vi "ECEF_2_LLA2(SubVI).vi"(11 "p_new":dbl[](array[numeric])) -> (1 "lon":dbl, 2 "latd":dbl, 3 "altd":dbl)   [LabVIEW 2017]
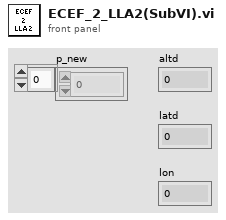
[diagram p1: front panel]
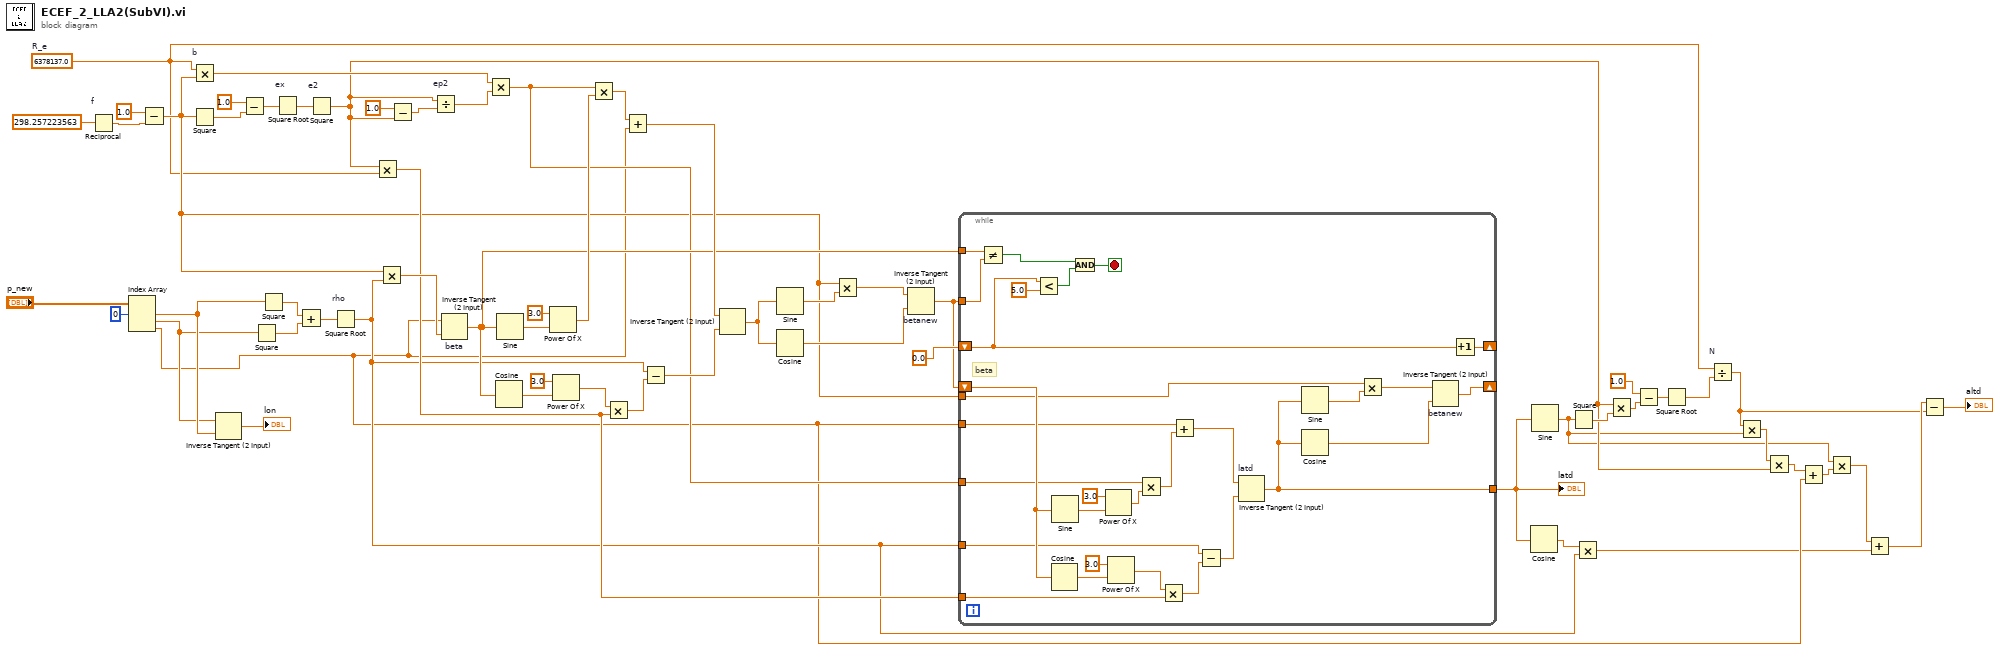
[diagram p0: block diagram]
diagram:
  w20 = 6378137.0  # R_e
  n1 = Reciprocal "f"(x=298.257223563) -> (1/x=w56:dbl)
  n2 = Index Array(array="p_new", index #1=0 ("index")) -> (element #1=w48:dbl, element #2=w47:dbl, element #3=w8:dbl)  [unwired: 2 in]
  n3 = Subtract(x=1.0, y=w56) -> (x-y=w21:dbl)
  n4 = Multiply "b"(x=w20, y=w21) -> (x*y=w42:dbl)
  n5 = Square(x=w21) -> (x^2=w54:dbl)
  n6 = Inverse Tangent (2 Input)(1:w48, 2:w47) -> (0:→"lon":dbl)
  n7 = Subtract(x=1.0, y=w54) -> (x-y=w53:dbl)
  n8 = Square(x=w47) -> (x^2=w45:dbl)
  n9 = Square(x=w48) -> (x^2=w46:dbl)
  n10 = Square Root "ex"(x=w53) -> (sqrt(x)=w52:dbl)
  n11 = Add(x=w46, y=w45) -> (x+y=w44:dbl)
  n12 = Square "e2"(x=w52) -> (x^2=w10:dbl)
  n13 = Square Root "rho"(x=w44) -> (sqrt(x)=w12:dbl)
  n14 = Multiply(x=w10, y=w20) -> (x*y=w22:dbl)
  n15 = Multiply(x=w21, y=w12) -> (x*y=w43:dbl)
  n16 = Subtract(x=1.0, y=w10) -> (x-y=w50:dbl)
  n17 = Divide "ep2"(x=w10, y=w50) -> (x/y=w41:dbl)
  n18 = Inverse Tangent (2 Input) "beta"(1:w43, 2:w8) -> (0:w26:dbl)
  n19 = Multiply(x=w42, y=w41) -> (x*y=w23:dbl)
  n20 = Cosine(x=w26) -> (cos(x)=w35:dbl)
  n21 = Sine(x=w26) -> (sin(x)=w40:dbl)
  n22 = Power Of X(1:w40, 2:3.0 ("y")) -> (0:w38:dbl)
  n23 = Power Of X(1:w35, 2:3.0 ("y")) -> (0:w34:dbl)
  n24 = Multiply(x=w23, y=w38) -> (x*y=w37:dbl)
  n25 = Multiply(x=w34, y=w22) -> (x*y=w33:dbl)
  n26 = Add(x=w37, y=w8) -> (x+y=w31:dbl)
  n27 = Subtract(x=w12, y=w33) -> (x-y=w32:dbl)
  n28 = Inverse Tangent (2 Input)(1:w32, 2:w31) -> (0:w30:dbl)
  n29 = Sine(x=w30) -> (sin(x)=w29:dbl)
  n30 = Cosine(x=w30) -> (cos(x)=w27:dbl)
  n31 = Multiply(x=w21, y=w29) -> (x*y=w28:dbl)
  n32 = Inverse Tangent (2 Input) "betanew"(1:w27, 2:w28) -> (0:w24:dbl)
  n33 = while {
    tunnel: w26 -> [w89]
    tunnel: w24 -> [w88]
    shift-right: [w84] -> _
    shift-left: 0.0 -> [w83]
    shift-right: [w62] -> _
    shift-left: w24 -> [w75]
    tunnel: w8 -> [w74]
    tunnel: w23 -> [w72]
    tunnel: w22 -> [w70]
    tunnel: w12 -> [w69]
    tunnel: [w63] -> w14
    tunnel: w21 -> [w61]
    stop <- w82 stop-if-true
    # "beta"
    n34 = Not Equal?(x=w89, y=w88) -> (x != y?=w87:bool)
    n35 = Less?(x=w83, y=5.0) -> (x < y?=w86:bool)
    n36 = Cosine(x=w75) -> (cos(x)=w78:dbl)
    n37 = Sine(x=w75) -> (sin(x)=w81:dbl)
    n38 = And(x=w87, y=w86) -> (x .and. y?=w82:bool)
    n39 = Power Of X(1:w81, 2:3.0 ("y")) -> (0:w73:dbl)
    n40 = Power Of X(1:w78, 2:3.0 ("y")) -> (0:w77:dbl)
    n41 = Multiply(x=w72, y=w73) -> (x*y=w71:dbl)
    n42 = Multiply(x=w77, y=w70) -> (x*y=w76:dbl)
    n43 = Add(x=w74, y=w71) -> (x+y=w68:dbl)
    n44 = Subtract(x=w69, y=w76) -> (x-y=w67:dbl)
    n45 = Inverse Tangent (2 Input) "latd"(1:w67, 2:w68) -> (0:w63:dbl)
    n46 = Sine(x=w63) -> (sin(x)=w66:dbl)
    n47 = Cosine(x=w63) -> (cos(x)=w64:dbl)
    n48 = Multiply(x=w61, y=w66) -> (x*y=w65:dbl)
    n49 = Inverse Tangent (2 Input) "betanew"(1:w64, 2:w65) -> (0:w62:dbl)
    n50 = Increment(x=w83) -> (x+1=w84:dbl)
  }
  "latd" <- w14
  n51 = Cosine(x=w14) -> (cos(x)=w13:dbl)
  n52 = Sine(x=w14) -> (sin(x)=w5:dbl)
  n53 = Square(x=w5) -> (x^2=w19:dbl)
  n54 = Multiply(x=w13, y=w12) -> (x*y=w7:dbl)
  n55 = Multiply(x=w10, y=w19) -> (x*y=w18:dbl)
  n56 = Subtract(x=1.0, y=w18) -> (x-y=w16:dbl)
  n57 = Square Root(x=w16) -> (sqrt(x)=w15:dbl)
  n58 = Divide "N"(x=w20, y=w15) -> (x/y=w2:dbl)
  n59 = Multiply(x=w2, y=w5) -> (x*y=w11:dbl)
  n60 = Multiply(x=w11, y=w10) -> (x*y=w9:dbl)
  n61 = Add(x=w9, y=w8) -> (x+y=w6:dbl)
  n62 = Multiply(x=w5, y=w6) -> (x*y=w4:dbl)
  n63 = Add(x=w4, y=w7) -> (x+y=w3:dbl)
  n64 = Subtract(x=w3, y=w2) -> (x-y=→"altd":dbl)
